vi "_CleanUp.vi"(8 "error in (no error)":errorcluster, 11 "MDPtrMgr in":refnum<class "MDPtrMgr.lvclass">) -> (0 "error out":errorcluster, 3 "MDPtrMgr out":refnum<class "MDPtrMgr.lvclass">)   [LabVIEW 2017, in "MDPtr.lvlib" / "MDPtrMgr.lvclass"]
uses:
  MDPtrMgr.lvclass
  MDPtrMgr.lvclass/MDPtrMgr.ctl
  MDPtr TypeDef/MDPtr DataFrame-Memory.ctl
  MDPtr TypeDef/MDPtr DataFrame-Common.ctl
  <vilib>/Utility/Data Type/Type Definitions/Data Type.ctl
  MDPtr.lvlib
  <vilib>/Utility/Data Type/NI_Data Type.lvlib
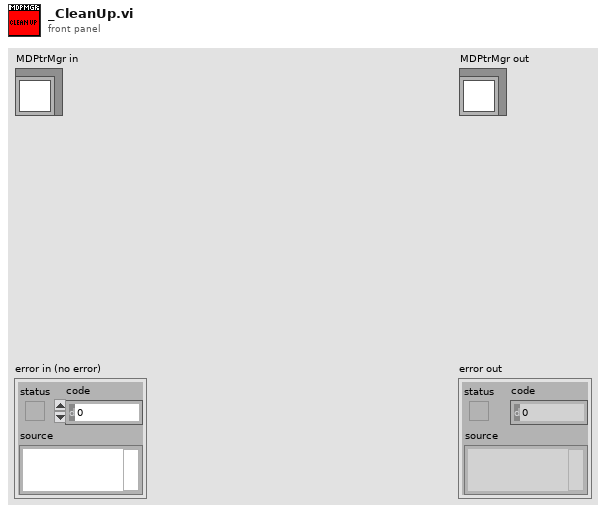
[diagram p1: front panel]
types:
  T1 = typedef "MDPtr.lvlib/MDPtr Queue.ctl" = refnum<queue>
  T2 = typedef "MDPtr.lvlib/MDPtr.ctl" = refnum<k1>
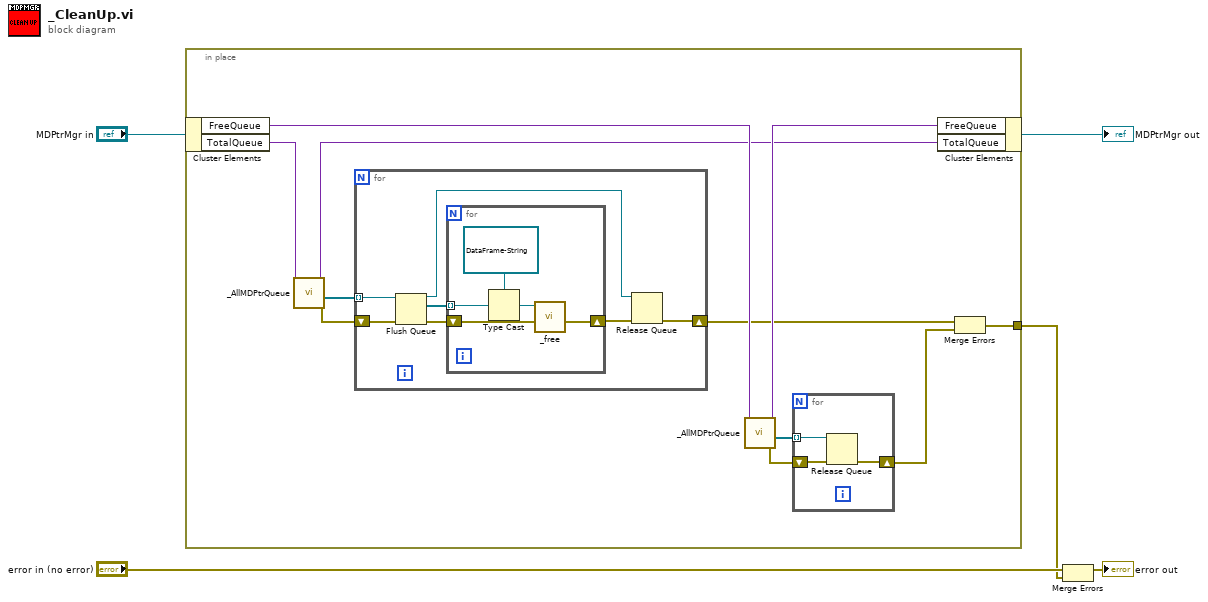
[diagram p0: block diagram]
diagram:
  n1 = in-place "In Place Element Structure" {
    in-place-border: [w6] -> w1
    n2 = in-place-cluster #1("MDPtrMgr in") -> ("FreeQueue"=w16:variant, "TotalQueue"=w14:variant)
    n3 = call "_AllMDPtrQueue.vi"("Variant in"=w14) -> ("error out"=w12:errorcluster, "Array"=w11:T1[], "Variant"=w13:variant)  [unwired: 8 in]
    n4 = for {
      tunnel: w11 -> [w26] mode=indexing
      shift-right: [w21] -> w8
      shift-left: w12 -> [w24]
      n5 = Flush Queue(queue=w26, error in (no error)=w24) -> (queue out=w20:T1, remaining elements=w25:T2[], error out=w23:errorcluster)
      n6 = for {
        tunnel: w25 -> [w29] mode=indexing
        shift-right: [w27] -> w22
        shift-left: w23 -> [w28]
        n7 = Type Cast(type=refnum<data-value> refnum ("MDPtr DVR"), x=w29) -> (*(type *) &x=w31:refnum<data-value>)
        n8 = call "_free.vi"("error in (no error)"=w28, "MDPtr DVR"=w31) -> ("error out"=w27:errorcluster)  [unwired: 8 in]
      }
      n9 = Release Queue(queue=w20, error in (no error)=w22) -> (error out=w21:errorcluster)  [unwired: 1 in, 2 out]
    }
    n10 = call "_AllMDPtrQueue.vi"("Variant in"=w16) -> ("error out"=w9:errorcluster, "Array"=w10:T1[], "Variant"=w15:variant)  [unwired: 8 in]
    n11 = for {
      shift-right: [w19] -> w7
      shift-left: w9 -> [w18]
      tunnel: w10 -> [w17] mode=indexing
      n12 = Release Queue(queue=w17, error in (no error)=w18) -> (error out=w19:errorcluster)  [unwired: 1 in, 2 out]
    }
    n13 = in-place-cluster #1("FreeQueue"=w15, "TotalQueue"=w13) -> (→"MDPtrMgr out":refnum<class "MDPtrMgr.lvclass">)
    n14 = Merge Errors(w8, w7) -> (w6:errorcluster)
  }
  n15 = Merge Errors("error in (no error)", w1) -> (→"error out":errorcluster)
